vi "Write ENG.vi"(8 "error in (no error)":errorcluster, 10 "ENG":bool, 11 "Coffee Actor in":refnum<class "Coffee Actor.lvclass">) -> (0 "error out":errorcluster, 3 "Coffee Actor out":refnum<class "Coffee Actor.lvclass">)   [LabVIEW 2019, in "Coffee Actor.lvlib" / "Coffee Actor.lvclass"]
uses:
  Coffee Actor.lvclass
  Coffee Actor.lvclass/Coffee Actor.ctl
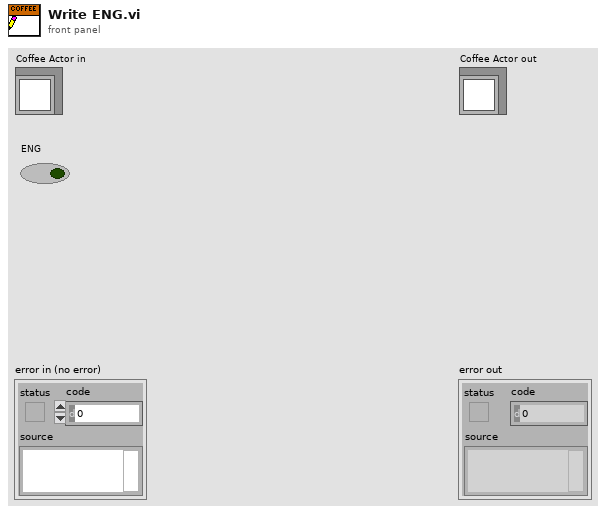
[diagram p1: front panel]
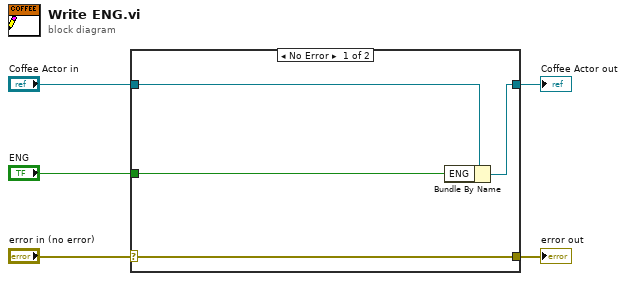
[diagram p0: block diagram]
diagram:
  n1 = case shown="No Error" "error in (no error)" {
    selector: "error in (no error)" -> [w9 w10]
    tunnel: [w9 w10] -> w4
    tunnel: [w7 w11] -> w2
    tunnel: "Coffee Actor in" -> [w8 w11]
    tunnel: "ENG" -> [w6 _]
    frame No Error {
      n2 = Bundle By Name(cluster=w8, "ENG"=w6) -> (w7:refnum<class "Coffee Actor.lvclass">)
    }
    frame Error {
    }
  }
  "error out" <- w4
  "Coffee Actor out" <- w2
